vi "Release Control Cluster.vi"(11 "output cluster":T1={"I-O.lvclass"=refnum, "Gantry"=refnum, "Dispenser"="COM1"}) -> ()   [LabVIEW 2021, in "Controller.lvclass"]
uses:
  Controller.lvclass
  Controllers.ctl
  I-O/I-O.lvclass
  C:/Program Files (x86)/Aerotech/A3200/LabVIEW/2010/Bin/Aerotech.A3200.dll
  Program Files (x86)/Aerotech/A3200/LabVIEW/2010/Bin/Aerotech.A3200.dll
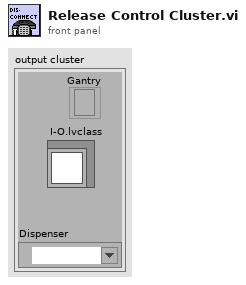
[diagram p1: front panel]
types:
  T1 = typedef "Controller.lvclass/Controllers.ctl" = cluster{"I-O.lvclass":refnum<class "I-O.lvclass">, "Gantry":refnum<k24>, "Dispenser":refnum<visa-resource-name>}
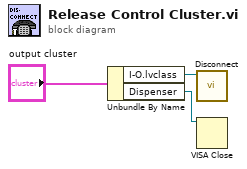
[diagram p0: block diagram]
diagram:
  n1 = Unbundle By Name("output cluster") -> ("I-O.lvclass"=w2:refnum<class "I-O.lvclass">, "Dispenser"=w1:refnum<visa-resource-name>)
  n2 = call-dynamic "Disconnect.vi"("I-O in"=w2) -> ()  [unwired: 9 in, 1 out]
  n3 = VISA Close(VISA resource name=w1) -> ()  [unwired: 1 in, 1 out]
